vi "WaveformNaming.vi"(1 "Waveform Name":string[](array[string]), 2 "Waveforms In":digitalwaveform[](graph)) -> (0 "Waveforms Out":digitalwaveform[](array[waveform]))   [LabVIEW 2016]
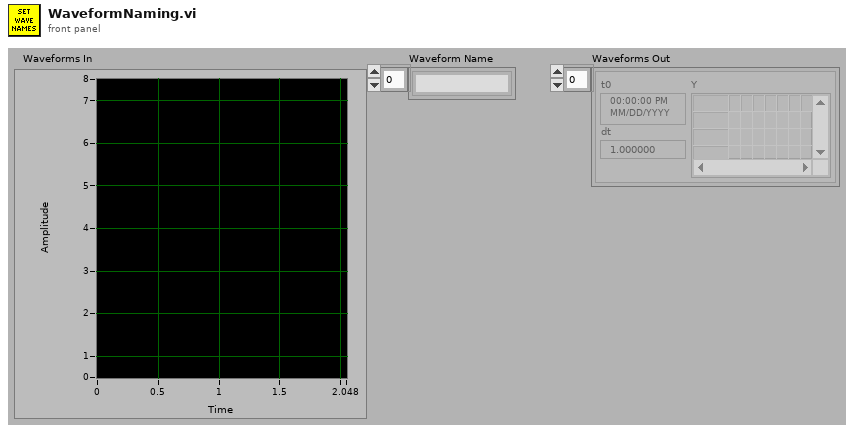
[diagram p1: front panel]
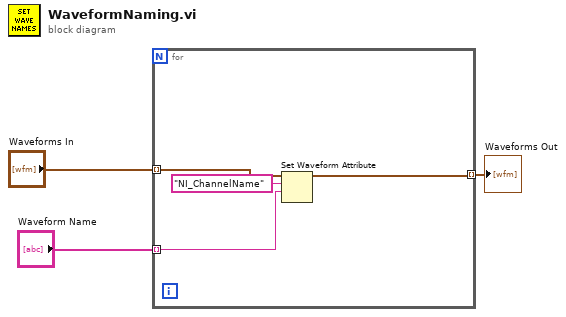
[diagram p0: block diagram]
diagram:
  n1 = for {
    tunnel: "Waveforms In" -> [w7] mode=indexing
    tunnel: "Waveform Name" -> [w6] mode=indexing
    tunnel: [w4] -> w1 mode=indexing
    n2 = Set Waveform Attribute(5:w6, 6:"NI_ChannelName" ("name"), 7:w7) -> (3:w4:digitalwaveform)  [unwired: 1 in, 2 out]
  }
  "Waveforms Out" <- w1
